vi "Sensor Setting.vi"(8 "error in":errorcluster) -> (0 "error  out":errorcluster)   [LabVIEW 2015]
uses:
  Control Button/Save.ctl
  Control Button/Exit.ctl
  Control Button/Delete.ctl
  <vilib>/addons/database/Connection.llb/DB Tools Open Connec (String).vi
  Galobal variable_TI.vi
  <vilib>/addons/database/_DB Variant To Data/Database Variant To Data.xnode
  <vilib>/addons/database/NI_Database_API.lvlib
panel:
  in  "Delete":T1
  out "error out":errorcluster
  out "columns":string[](array[string])
  in  "String":string
  out "Load (N)":dbl format="%0.03f"
  in  "Setting Data":T2 {"Load Offset" format="%0.03f"; "MaxLoad(N)" format="%0.02f"; "Min Load(N)" format="%0.02f"}
  out "Model":string
  in  "Select Model":string(combo)
  in  "Exit":T3
  in  "Save":T4
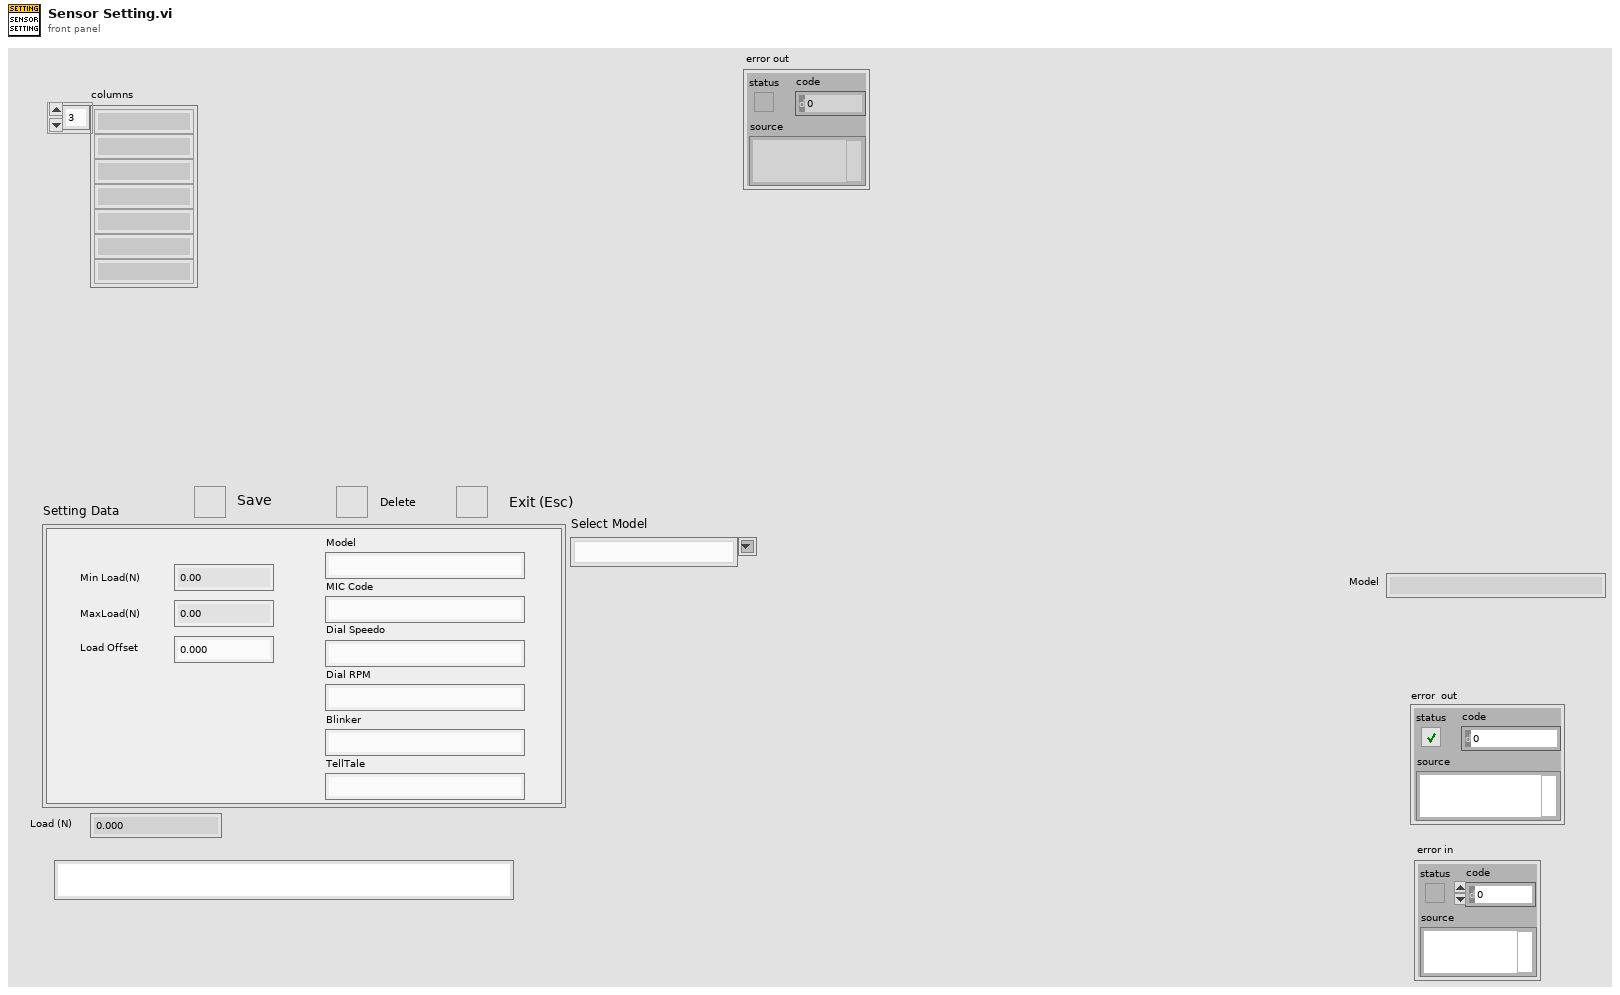
[diagram p1: front panel]
types:
  T1 = typedef "Delete.ctl" = bool
  T2 = cluster{"MaxLoad(N) ":dbl, "Min Load(N)":dbl, "Load Offset":dbl, "Model":string, "MIC Code":string, "Dial Speedo":string, "Dial RPM":string, "Blinker":string, "TellTale":string}
  T3 = typedef "Exit.ctl" = bool
  T4 = typedef "Save.ctl" = bool
  T5 = cluster{"MaxLoad(N) ":dbl, "Min Load(N)":dbl, "Load Offset":dbl, "Model":string, "MIC Code":string, "Dailcode1":string, "Dailcode2":string, "DailStrip1":string, "DailStrip2":string}
  T6 = typedef "NI_Database_API.lvlib/Conn ObjectReference.ctl" = refnum<k1>
  T7 = enum16{"Left Button", "Center Button", "Right Button", "Window Close"}
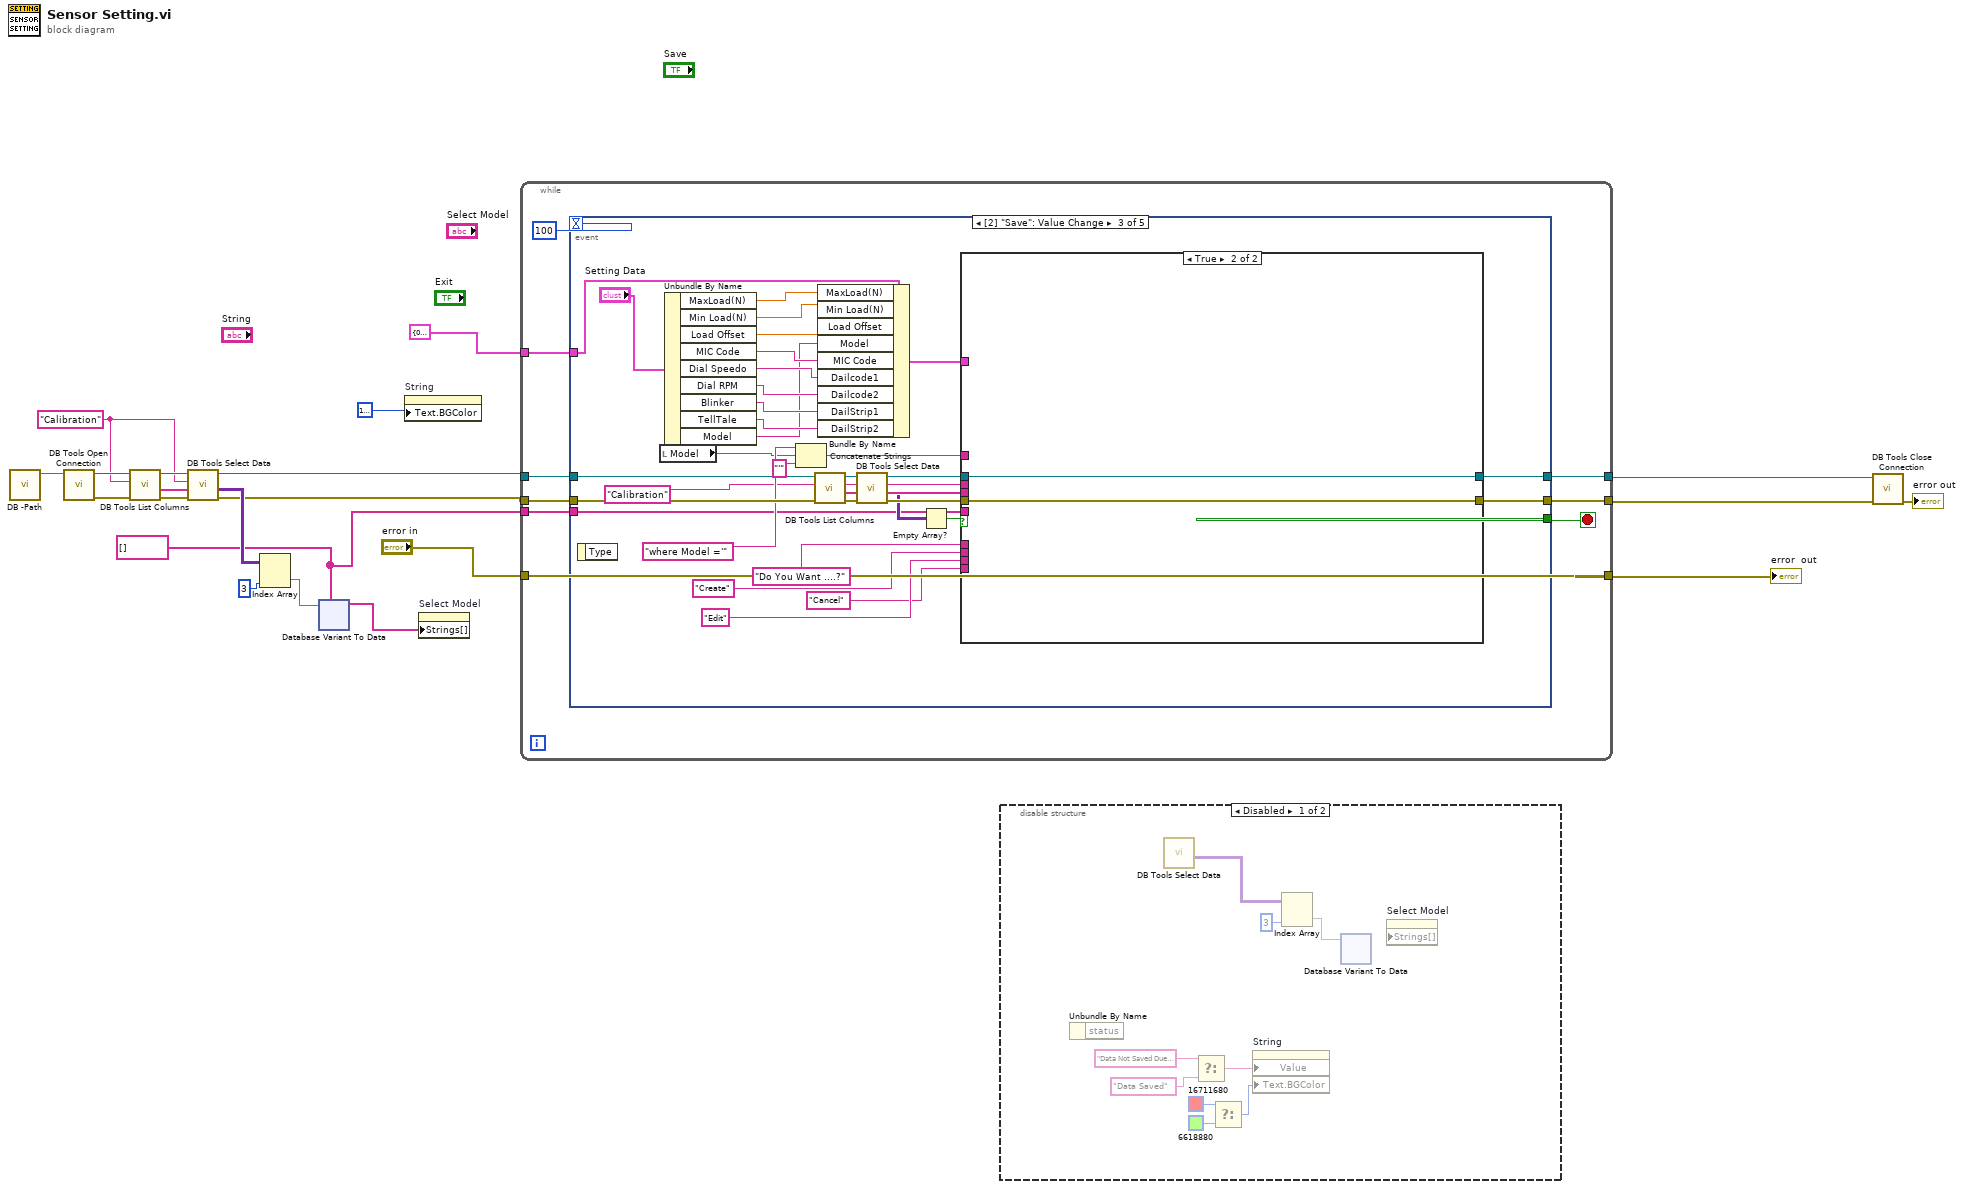
[diagram p0: block diagram]
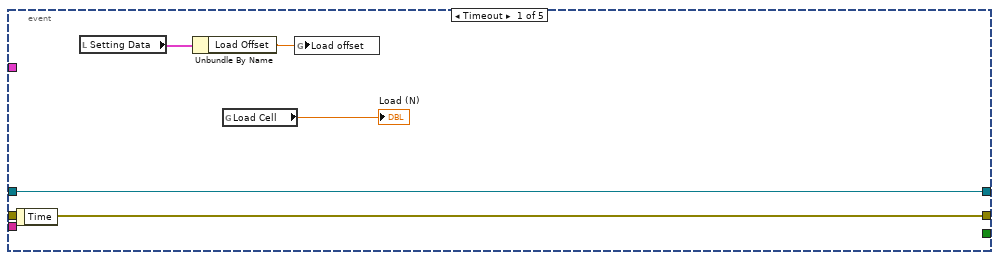
[diagram p3: hidden frame]
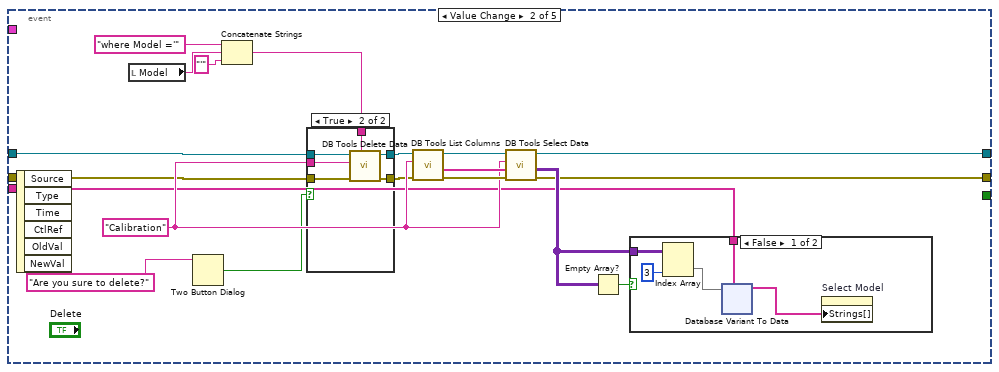
[diagram p4: hidden frame]
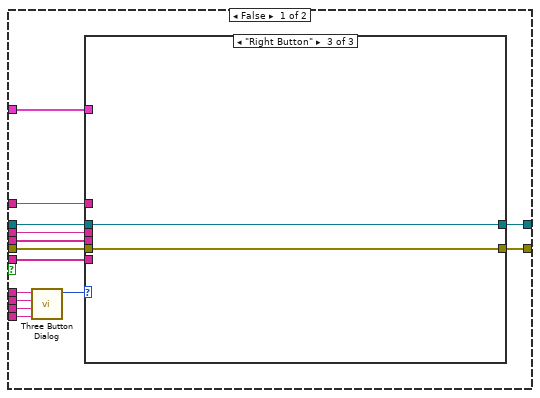
[diagram p7: hidden frame]
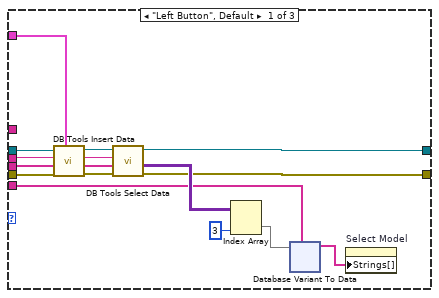
[diagram p8: hidden frame]
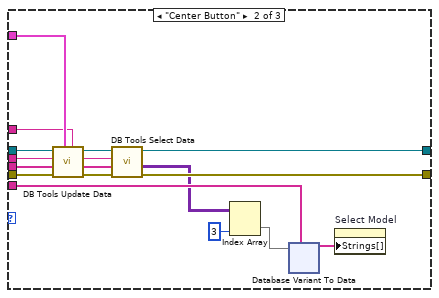
[diagram p9: hidden frame]
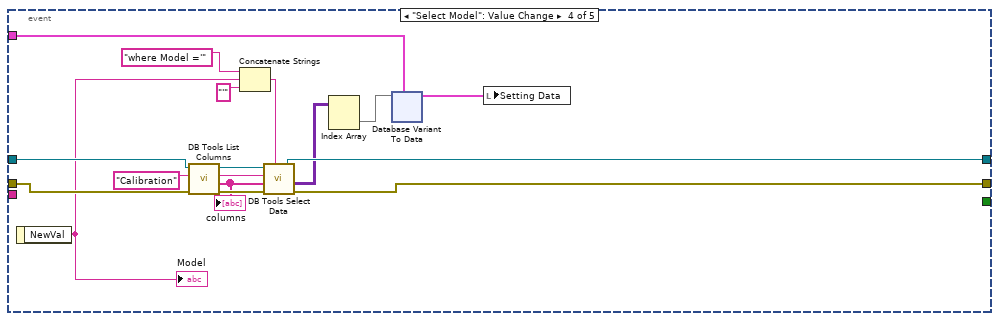
[diagram p10: hidden frame]
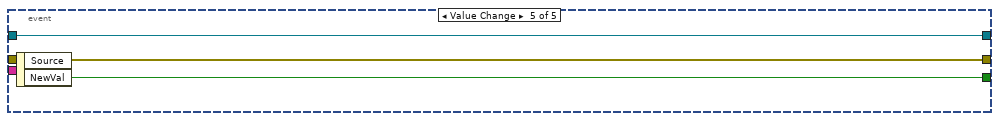
[diagram p11: hidden frame]
diagram:
  w1 = string[] [] ("Programlist")
  w9 = "Calibration" ("table")
  n1 = call "DB -Path.vi"() -> ("String"=w21:string)  [unwired: 11 in]
  n2 = call-poly <vilib>:"DB Tools Open Connection.vi"("connection information"=w21) -> ("error out"=w13:errorcluster, "connection reference"=w12:T6)  [unwired: 7 in]
  n3 = call <vilib>:"DB Tools List Columns.vi"("error in (no error)"=w13, "table"=w9, "connection reference"=w12) -> ("error out"=w10:errorcluster, "columns"=w8:string[], "connection reference out"=w11:T6)  [unwired: 1 in, 1 out]
  n4 = call <vilib>:"DB Tools Select Data.vi"("error in (no error)"=w10, "columns"=w8, "table"=w9, "connection reference"=w11) -> ("error out"=w5:errorcluster, "data"=w7:variant[][], "connection reference out"=w6:T6)  [unwired: 2 in]
  n5 = Index Array(array=w7, index (col)=3 ("disabled index (col)")) -> (element=w4:variant[])  [unwired: 1 in]
  n6 = xnode "Database Variant To Data"("database variant"=w4, "type"=w1) -> ("data"=w2:string[])  [unwired: 1 in, 1 out]
  n7 = property on="String" class="Str"("Text.BGColor"=u32 16777226 ("Color Box")) -> ()  [unwired: 2 in, 2 out]
  n8 = property on="Select Model" class="CmbBox"("Strings[]"=w2) -> ()  [unwired: 2 in, 2 out]
  n9 = while {
    tunnel: w6 -> [w29]
    tunnel: w5 -> [w28]
    tunnel: [w27] -> w20
    tunnel: [w26] -> w19
    tunnel: "error in" -> [w24]
    tunnel: [w24] -> w17
    tunnel: T5 {"MaxLoad(N) "=0.0, "Min Load(N)"=0.0, "Load Offset"=0.0, "Model"="", "MIC Code"="", "Dailcode1"="", "Dailcode2"="", "DailStrip1"="", "DailStrip2"=""} ("Setting Data") -> [w23]
    tunnel: w1 -> [w22]
    stop <- w25 stop-if-true
    n10 = event shown="[2] \"Save\": Value Change" {
      selector: _ -> [_ _ _ _ _]
      dyn-events: _ -> [_ _ _ _ _]
      timeout: 100 -> [_ _ _ _ _]
      tunnel: w29 -> [w35 w46 w138 w270 w562]
      tunnel: w28 -> [w34 w47 w137 w269 w563]
      tunnel: [w35 w40 w108 w268 w562] -> w27
      tunnel: [w34 w39 w107 w267 w563] -> w26
      tunnel: [_ _ _ _ w561] -> w25
      tunnel: w23 -> [_ _ w131 w264 _]
      tunnel: w22 -> [_ w42 w109 _ _]
      event Timeout {
        n11 = event-data() -> ()  [unwired: 1 in, 1 out]
        n12 = local read "Setting Data"() -> (w32:T2)
        n13 = Unbundle By Name(w32) -> ("Load Offset"=w31:dbl)
        n14 = global read "Galobal variable_TI.vi" "Load Cell"() -> (→"Load (N)":dbl)
        n15 = global write "Galobal variable_TI.vi" "Load offset"(w31) -> ()
      }
      event Value Change {
        w48 = "Calibration" ("table")
        n16 = event-data() -> ()  [unwired: 1 in, 6 out]
        n17 = local read "Model"() -> (w50:string)
        n18 = Two Button Dialog(message="Are you sure to delete?") -> (T button?=w37:bool)  [unwired: 2 in]
        n19 = Concatenate Strings("where Model ='" ("string"), w50, "'" ("string")) -> (w49:string)
        n20 = case shown="True" w37 {
          tunnel: w49 -> [_ w62]
          tunnel: w48 -> [_ w61]
          tunnel: w47 -> [w55 w60]
          tunnel: w46 -> [w56 w59]
          tunnel: [w56 w58] -> w45
          tunnel: [w55 w57] -> w44
          frame False {
          }
          frame True {
            n21 = call <vilib>:"DB Tools Delete Data.vi"("condition"=w62, "error in (no error)"=w60, "table"=w61, "connection reference"=w59) -> ("error out"=w57:errorcluster, "connection reference out"=w58:T6)  [unwired: 6 in]
          }
        }
        n22 = call <vilib>:"DB Tools List Columns.vi"("error in (no error)"=w44, "table"=w48, "connection reference"=w45) -> ("error out"=w54:errorcluster, "columns"=w53:string[], "connection reference out"=w38:T6)  [unwired: 1 in, 1 out]
        n23 = call <vilib>:"DB Tools Select Data.vi"("error in (no error)"=w54, "columns"=w53, "table"=w48, "connection reference"=w38) -> ("error out"=w39:errorcluster, "data"=w43:variant[][], "connection reference out"=w40:T6)  [unwired: 2 in]
        n24 = Empty Array?(array=w43) -> (empty?=w41:bool)
        n25 = case shown="False" w41 {
          tunnel: w43 -> [w64 _]
          tunnel: w42 -> [w63 _]
          frame False {
            n26 = Index Array(array=w64, index (col)=3 ("disabled index (col)")) -> (element=w65:variant[])  [unwired: 1 in]
            n27 = xnode "Database Variant To Data"("database variant"=w65, "type"=w63) -> ("data"=w67:string[])  [unwired: 1 in, 1 out]
            n28 = property on="Select Model" class="CmbBox"("Strings[]"=w67) -> ()  [unwired: 2 in, 2 out]
          }
          frame True {
          }
        }
      }
      event Value Change {
        w120 = "Calibration" ("table")
        n29 = event-data() -> ()  [unwired: 1 in, 1 out]
        n30 = local read "Model"() -> (w132:string)
        n31 = Unbundle By Name("Setting Data") -> ("MaxLoad(N)"=w129:dbl, "Min Load(N)"=w128:dbl, "Load Offset"=w127:dbl, "MIC Code"=w126:string, "Dial Speedo"=w125:string, "Dial RPM"=w124:string, "Blinker"=w123:string, "TellTale"=w122:string, "Model"=w106:string)
        n32 = Concatenate Strings("where Model ='" ("string"), w132, "'" ("string")) -> (w133:string)
        n33 = call <vilib>:"DB Tools List Columns.vi"("error in (no error)"=w137, "table"=w120, "connection reference"=w138) -> ("error out"=w121:errorcluster, "columns"=w119:string[], "connection reference out"=w117:T6)  [unwired: 1 in, 1 out]
        n34 = Bundle By Name(cluster=w131, "MaxLoad(N)"=w129, "Min Load(N)"=w128, "Load Offset"=w127, "Model"=w106, "MIC Code"=w126, "Dailcode1"=w125, "Dailcode2"=w124, "DailStrip1"=w123, "DailStrip2"=w122) -> (w136:T5)
        n35 = call <vilib>:"DB Tools Select Data.vi"("error in (no error)"=w121, "columns"=w119, "table"=w120, "connection reference"=w117) -> ("error out"=w118:errorcluster, "data"=w115:variant[][], "connection reference out"=w116:T6)  [unwired: 2 in]
        n36 = Empty Array?(array=w115) -> (empty?=w114:bool)
        n37 = case shown="True" w114 {
          tunnel: w118 -> [w152 w260]
          tunnel: w116 -> [w151 w261]
          tunnel: w119 -> [w150 _]
          tunnel: w136 -> [w149 _]
          tunnel: w133 -> [w148 _]
          tunnel: w120 -> [w147 _]
          tunnel: "Do You Want ....?" ("message") -> [w146 _]
          tunnel: "Create" ("Left Button Text (\"Yes\")") -> [w145 _]
          tunnel: "Edit" ("Center Button Text (\"No\")") -> [w144 _]
          tunnel: "Cancel" ("Right Button Text (\"Cancel\")") -> [w143 _]
          tunnel: w109 -> [w141 _]
          tunnel: [w140 w261] -> w108
          tunnel: [w139 w260] -> w107
          frame False {
            n38 = call <vilib>:"Three Button Dialog.vi"("Right Button Text (\"Cancel\")"=w143, "Center Button Text (\"No\")"=w144, "Left Button Text (\"Yes\")"=w145, "message"=w146) -> ("Which Button?"=w142:T7)  [unwired: 7 in]
            n39 = case shown="\"Right Button\"" w142 {
              tunnel: w152 -> [w159 w219 w258]
              tunnel: w151 -> [w160 w218 w259]
              tunnel: w150 -> [w157 w208 _]
              tunnel: w149 -> [w156 w217 _]
              tunnel: w148 -> [_ w216 _]
              tunnel: w147 -> [w158 w209 _]
              tunnel: w141 -> [w161 w212 _]
              tunnel: [w155 w207 w259] -> w140
              tunnel: [w154 w206 w258] -> w139
              frame "Left Button", Default {
                n40 = call <vilib>:"DB Tools Insert Data.vi"("data"=w156, "error in (no error)"=w159, "columns"=w157, "table"=w158, "connection reference"=w160) -> ("error out"=w163:errorcluster, "connection reference out"=w164:T6)  [unwired: 5 in]
                n41 = call <vilib>:"DB Tools Select Data.vi"("error in (no error)"=w163, "columns"=w157, "table"=w158, "connection reference"=w164) -> ("error out"=w154:errorcluster, "data"=w162:variant[][], "connection reference out"=w155:T6)  [unwired: 2 in]
                n42 = Index Array(array=w162, index (col)=3 ("disabled index (col)")) -> (element=w165:variant[])  [unwired: 1 in]
                n43 = xnode "Database Variant To Data"("database variant"=w165, "type"=w161) -> ("data"=w153:string[])  [unwired: 1 in, 1 out]
                n44 = property on="Select Model" class="CmbBox"("Strings[]"=w153) -> ()  [unwired: 2 in, 2 out]
              }
              frame "Center Button" {
                n45 = call <vilib>:"DB Tools Update Data.vi"("condition"=w216, "data"=w217, "error in (no error)"=w219, "columns"=w208, "table"=w209, "connection reference"=w218) -> ("error out"=w210:errorcluster, "connection reference out"=w211:T6)  [unwired: 4 in]
                n46 = call <vilib>:"DB Tools Select Data.vi"("error in (no error)"=w210, "columns"=w208, "table"=w209, "connection reference"=w211) -> ("error out"=w206:errorcluster, "data"=w205:variant[][], "connection reference out"=w207:T6)  [unwired: 2 in]
                n47 = Index Array(array=w205, index (col)=3 ("disabled index (col)")) -> (element=w214:variant[])  [unwired: 1 in]
                n48 = xnode "Database Variant To Data"("database variant"=w214, "type"=w212) -> ("data"=w213:string[])  [unwired: 1 in, 1 out]
                n49 = property on="Select Model" class="CmbBox"("Strings[]"=w213) -> ()  [unwired: 2 in, 2 out]
              }
              frame "Right Button" {
              }
            }
          }
          frame True {
          }
        }
      }
      event "Select Model": Value Change {
        w271 = "Calibration" ("table")
        n50 = event-data() -> ("NewVal"=w262:string)  [unwired: 1 in]
        "Model" <- w262
        n51 = call <vilib>:"DB Tools List Columns.vi"("error in (no error)"=w269, "table"=w271, "connection reference"=w270) -> ("error out"=w277:errorcluster, "columns"=w275:string[], "connection reference out"=w276:T6)  [unwired: 1 in, 1 out]
        "columns" <- w275
        n52 = Concatenate Strings("where Model ='" ("string"), w262, "'" ("string")) -> (w272:string)
        n53 = call <vilib>:"DB Tools Select Data.vi"("condition"=w272, "error in (no error)"=w277, "columns"=w275, "table"=w271, "connection reference"=w276) -> ("error out"=w267:errorcluster, "data"=w266:variant[][], "connection reference out"=w268:T6)  [unwired: 1 in]
        n54 = Index Array(array=w266) -> (element=w265:variant[])  [unwired: 2 in]
        n55 = xnode "Database Variant To Data"("database variant"=w265, "type"=w264) -> ("data"=w263:T5)  [unwired: 1 in, 1 out]
        n56 = local write "Setting Data"(w263) -> ()
      }
      event Value Change {
        n57 = event-data() -> ("NewVal"=w561:T3)  [unwired: 1 in, 1 out]
      }
    }
  }
  "error  out" <- w17
  n58 = disable-structure shown="Disabled" {
    frame Disabled {
      n59 = Unbundle By Name() -> ()  [unwired: 1 in, 1 out]
      n60 = call <vilib>:"DB Tools Select Data.vi"() -> ("data"=w566:variant[][])  [unwired: 6 in, 2 out]
      n61 = Select(t="Data Not Saved Due to Error In Database", f="Data Saved") -> (s? t:f=w570:string)  [unwired: 1 in]
      n62 = Select(t=u32 16711680 ("Color Box"), f=u32 6618880 ("Color Box")) -> (s? t:f=w572:u32)  [unwired: 1 in]
      n63 = property on="String" class="Str"("Value"=w570, "Text.BGColor"=w572) -> ()  [unwired: 2 in, 2 out]
      n64 = Index Array(array=w566, index (col)=3 ("disabled index (col)")) -> (element=w565:variant[])  [unwired: 1 in]
      n65 = xnode "Database Variant To Data"("database variant"=w565) -> ()  [unwired: 2 in, 2 out]
      n66 = property on="Select Model" class="CmbBox" props=["Strings[]"]() -> ()  [unwired: 3 in, 2 out]
    }
    frame Enabled {
    }
  }
  n67 = call <vilib>:"DB Tools Close Connection.vi"("error in (no error)"=w19, "connection reference"=w20) -> ("error out"=→"error out":errorcluster)  [unwired: 5 in]
